vi "Open.vi"(8 "error in (no error)":errorcluster) -> (0 "error out":errorcluster, 3 "Handle":u32)   [LabVIEW 2016, in "Photon Counter.lvlib" / "C8855-01.lvlib"]
doc: "Resets the driver and acquires a handle to control this unit. The acquired handle is used to access this unit. Use this function when controlling only one C8855-01.\n\n\n\nHANDLE C8855API __stdcall C8855Open( void );"
uses:
  C8855-01.lvlib
  C8855-01api.dll
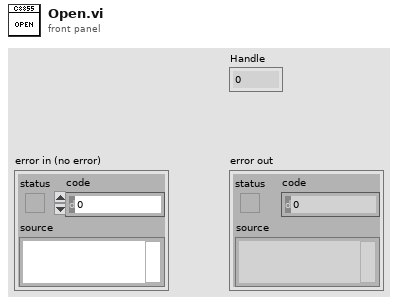
[diagram p1: front panel]
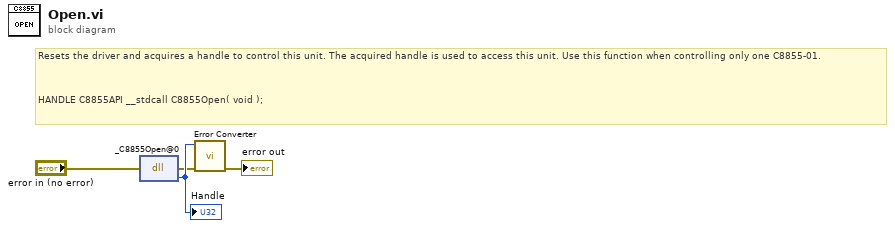
[diagram p0: block diagram]
diagram:
  # "Resets the driver and acquires a handle to control this unit. The acquired handle is used to access this unit. Use this function when controlling only one C8855-01.\n\n\n\nHANDLE C8855API __stdcall C8855Open( void );"
  n1 = dll-call lib="C:/Users/Andy/Desktop/Trace Grabber/Drivers/C8855-01/C8855-01api.dll" fn="_C8855Open@0"(error in="error in (no error)") -> (error out=w2:errorcluster, "return type"=w4:u32)  [unwired: 2 in, 1 out]
  "Handle" <- w4
  n2 = call "Error Converter.vi"("error in (no error)"=w2, "error code"=w4) -> ("error out"=→"error out":errorcluster)  [unwired: 9 in]
